vi "Open Hardware.vi"(8 "error in (no error)":errorcluster, 11 "Instrument.Aerotech in":refnum<class "Instrument.Aerotech.lvclass">) -> (0 "error out":errorcluster, 3 "Instrument.Aerotech out":refnum<class "Instrument.Aerotech.lvclass">)   [LabVIEW 2019, in "Instrument.Aerotech.lvclass"]
uses:
  Instrument.Aerotech.lvclass
  Instrument.Aerotech.lvclass/Instrument.Aerotech.ctl
  Aerotech-Ensemble-LabVIEW/2010-5.6/Motion/EnableSingle.vi
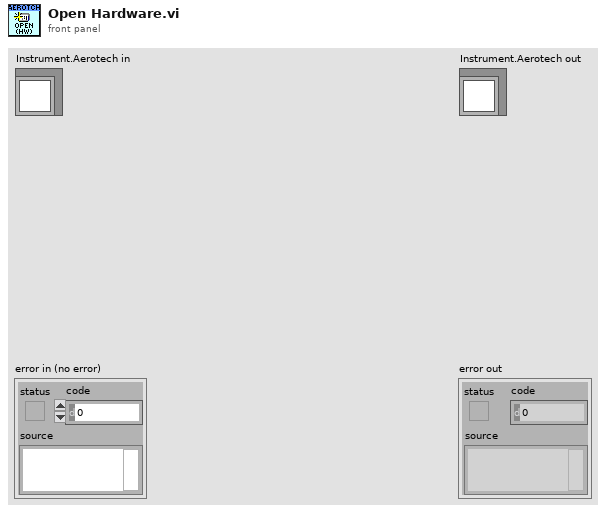
[diagram p1: front panel]
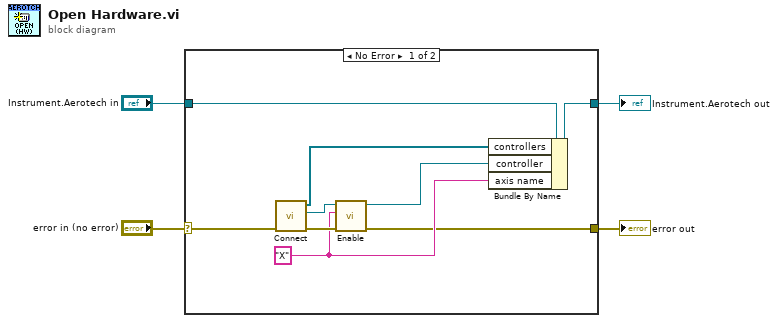
[diagram p0: block diagram]
diagram:
  n1 = case shown="No Error" "error in (no error)" {
    selector: "error in (no error)" -> [w5 w15]
    tunnel: "Instrument.Aerotech in" -> [w8 w14]
    tunnel: [w7 w14] -> w3
    tunnel: [w6 w15] -> w2
    frame No Error {
      w9 = "X" ("axis name")
      n2 = call "Connect.vi"("error in (no error)"=w5) -> ("error out"=w13:errorcluster, "controller"=w12:refnum<k24>, "controllers"=w11:refnum<k24>[])  [unwired: 8 in]
      n3 = call-poly "Enable.vi"("error in (no error)"=w13, "axis name"=w9, "controller in"=w12) -> ("error out"=w6:errorcluster, "controller out"=w10:refnum<k24>)  [unwired: 7 in]
      n4 = Bundle By Name(cluster=w8, "controllers"=w11, "controller"=w10, "axis name"=w9) -> (w7:refnum<class "Instrument.Aerotech.lvclass">)
    }
    frame Error {
    }
  }
  "error out" <- w2
  "Instrument.Aerotech out" <- w3
